vi "Single Character Display.vi"() -> ()   [LabVIEW 2014]
uses:
  <vilib>/myRIO/Instrument Drivers/Onboard IO/DIO/typedefs/DIO Reference.ctl
  <vilib>/myRIO/Common/Instrument Driver Framework/Utilities/typedefs/myRIO Generic Hardware Reference.ctl
  <vilib>/myRIO/Common/Instrument Driver Framework/Utilities/typedefs/Hardware Version Enum.ctl
  <vilib>/myRIO/Common/Instrument Driver Framework/Utilities/typedefs/myRIO v1.0 Reference.ctl
  <vilib>/myRIO/Common/Instrument Driver Framework/Utilities/typedefs/Generic FPGA Reference.ctl
  <vilib>/myRIO/Common/Instrument Driver Framework/myRIO v1.0/DIO/typedefs/DIO Channels List.ctl
  <vilib>/myRIO/Common/Instrument Driver Framework/myRIO v1.0/DIO/typedefs/DIO Channels Enum.ctl
  <vilib>/userdefined/High Color/nirio_resource_hc.ctl
  <vilib>/myRIO/Common/Instrument Driver Framework/Utilities/vis/Is FPGA Ref Available.vi
  <vilib>/myRIO/Common/Instrument Driver Framework/myRIO v1.0/DIO/vis/myRIO v1.1 Open DIO.vi
  <vilib>/myRIO/Instrument Drivers/Onboard IO/DIO/vis/Write.vi
  <vilib>/myRIO/Common/Instrument Driver Framework/Utilities/vis/Validate Channels.vi
  <vilib>/myRIO/Common/Instrument Driver Framework/myRIO v1.0/DIO/vis/myRIO v1.0 Reserve DIO.vi
  <vilib>/myRIO/Common/Instrument Driver Framework/myRIO v1.0/Resource Manager/vis/myRIO v1.0 Reserve Channel List.vi
  <vilib>/myRIO/Common/Instrument Driver Framework/myRIO v1.0/DIO/vis/myRIO v1.0 Build MUX Configuration DIO.vi
  <vilib>/myRIO/Common/Instrument Driver Framework/myRIO v1.0/Resource Manager/vis/myRIO v1.0 Reserve Channel.vi
  <vilib>/myRIO/Common/Instrument Driver Framework/myRIO v1.0/Resource Manager/vis/myRIO v1.0 Unreserve Channel.vi
  <vilib>/myRIO/Common/Instrument Driver Framework/myRIO v1.0/Resource Manager/vis/myRIO v1.0 Create Configuration List.vi
  <vilib>/myRIO/Common/Instrument Driver Framework/myRIO v1.0/Resource Manager/vis/myRIO v1.0 Build Mutex Name.vi
  <vilib>/Utility/VariantDataType/GetNumericInfo.vi
  <vilib>/Utility/error.llb/Error Cluster From Error Code.vi
  <vilib>/myRIO/Common/Instrument Driver Framework/myRIO v1.0/myRIO v1.1 Open.vi
  <vilib>/myRIO/Common/Instrument Driver Framework/Utilities/vis/IO Manager.vi
  <vilib>/myRIO/Common/Instrument Driver Framework/Utilities/vis/Configuration Manager.vi
  <vilib>/myRIO/Common/Instrument Driver Framework/myRIO v1.0/Resource Manager/vis/myRIO v1.0 Configure IO.vi
  <vilib>/myRIO/Common/Instrument Driver Framework/myRIO v1.0/myRIO v1.0 Close.vi
  <vilib>/myRIO/Common/Instrument Driver Framework/myRIO v1.0/DIO/vis/myRIO v1.0 Write DIO.vi
  <vilib>/myRIO/Express VI/Onboard IO/DO/DO Express VI.xnode
  <vilib>/myRIO/Instrument Drivers/Onboard IO/DIO/vis/myRIO DIO Open.xnode
  <vilib>/myRIO/Instrument Drivers/Onboard IO/DIO/DIO.lvlib
panel:
  out "Ones":bool[](array[boolean])
  out "Tens":bool[](array[boolean]) caption="Seconds"
  in  "Stop Button":bool
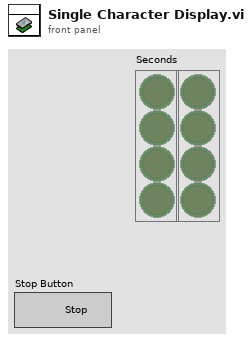
[diagram p1: front panel]
types:
  T1 = typedef "DIO.lvlib/DIO Reference.ctl" = cluster{"myRIO Reference":T2, "DIO Channels List":T6}
  T2 = typedef "myRIO Generic Hardware Reference.ctl" = cluster{"myRIO Model":T3, "myRIO Hardware Reference":T4}
  T3 = typedef "Hardware Version Enum.ctl" = enum16{"Unknown", "myRIO-1900", "myRIO-1950"}
  T4 = typedef "myRIO v1.0 Reference.ctl" = cluster{"Generic FPGA Reference":T5, "Allow multiple opens":bool}
  T5 = typedef "Generic FPGA Reference.ctl" = refnum<k20>
  T6 = typedef "DIO Channels List.ctl" = T7[]
  T7 = typedef "DIO Channels Enum.ctl" = enum16{"Not Connected", "C/DIO0", "C/DIO1", "C/DIO2", "C/DIO3", "C/DIO4", "C/DIO5", "C/DIO6", "C/DIO7", "A/DIO0", "A/DIO1", "A/DIO2", "A/DIO3", "A/DIO4", "A/DIO5", "A/DIO6", "A/DIO7", "A/DIO8", "A/DIO9", "A/DIO10", "A/DIO11", "A/DIO12", "A/DIO13", "A/DIO14", "A/DIO15", "B/DIO0", "B/DIO1", "B/DIO2", "B/DIO3", "B/DIO4", "B/DIO5", "B/DIO6", "B/DIO7", "B/DIO8", "B/DIO9", "B/DIO10", "B/DIO11", "B/DIO12", "B/DIO13", "B/DIO14", "B/DIO15", "LED0", "LED1", "LED2", "LED3", "Button0"}
  T8 = typedef "nirio_resource_hc.ctl" = tag
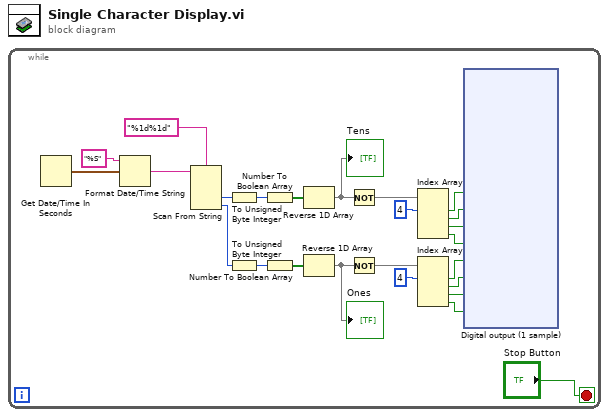
[diagram p0: block diagram]
diagram:
  n1 = while {
    stop <- "Stop Button" stop-if-true
    n2 = Get Date/Time In Seconds() -> (seconds since 1Jan1904=w5:timestamp)
    n3 = Format Date/Time String(time format string (%c)="%S", seconds (now)=w5) -> (date/time string=w4:string)  [unwired: 1 in]
    n4 = Scan From String(format string="%1d%1d", input string=w4) -> (output 1=w3:i32, output 2=w2:i32)  [unwired: 4 in, 3 out]
    n5 = To Unsigned Byte Integer(number=w3) -> (unsigned 8bit integer=w22:u8)
    n6 = To Unsigned Byte Integer(number=w2) -> (unsigned 8bit integer=w21:u8)
    n7 = Number To Boolean Array(number=w22) -> (Boolean array=w24:bool[])
    n8 = Number To Boolean Array(number=w21) -> (Boolean array=w23:bool[])
    n9 = Reverse 1D Array(array=w24) -> (reversed array=w20:bool[])
    "Tens" <- w20
    n10 = Reverse 1D Array(array=w23) -> (reversed array=w13:bool[])
    "Ones" <- w13
    n11 = Not(x=w20) -> (.not. x?=w8:bool[])
    n12 = Not(x=w13) -> (.not. x?=w7:bool[])
    n13 = Index Array(array=w8, index #1=4 ("index")) -> (element #1=w19:bool, element #2=w18:bool, element #3=w17:bool, element #4=w16:bool)  [unwired: 3 in]
    n14 = Index Array(array=w7, index #1=4 ("index")) -> (element #1=w15:bool, element #2=w14:bool, element #3=w12:bool, element #4=w11:bool)  [unwired: 3 in]
    n15 = xnode "Digital output (1 sample)"("B/DIO0 (Pin 11)"=w19, "B/DIO1 (Pin 13)"=w18, "B/DIO2 (Pin 15)"=w17, "B/DIO3 (Pin 17)"=w16, "B/DIO4 (Pin 19)"=w15, "B/DIO5 (Pin 21)"=w14, "B/DIO6 (Pin 23)"=w12, "B/DIO7 (Pin 25)"=w11) -> ()  [unwired: 1 in, 1 out]
  }
